vi "Cleanup.vi"(11 "asset utilization":refnum<class "NI SystemLink Asset Utilization.lvclass">) -> ()   [LabVIEW 2019]
uses:
  <vilib>/Skyline/AssetManagement/NI SystemLink Asset Utilization.lvclass
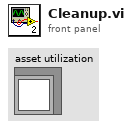
[diagram p1: front panel]
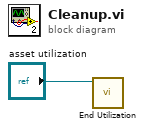
[diagram p0: block diagram]
diagram:
  n1 = call <vilib>:"End Utilization.vi"("asset utilization"="asset utilization") -> ()  [unwired: 10 in, 1 out]
